vi "Test Switch Tables 2.vi"() -> ()   [LabVIEW 2019]
uses:
  src/LV-Data.PG/LV-Data.PGSQL.lvclass
  <vilib>/addons/_JKI Toolkits/Caraya/classes/Test/Test.lvclass
  <vilib>/addons/_JKI Toolkits/Caraya/classes/Assert/Assert.lvclass
  <vilib>/addons/_JKI Toolkits/Caraya/classes/Assert/Assert Not Error.vi
panel:
  out "error out":errorcluster
  in  "error in (no error)":errorcluster
  out "Data.PG out":refnum<class "LV-Data.PGSQL.lvclass">
  in  "Data.PG":refnum<class "LV-Data.PGSQL.lvclass">
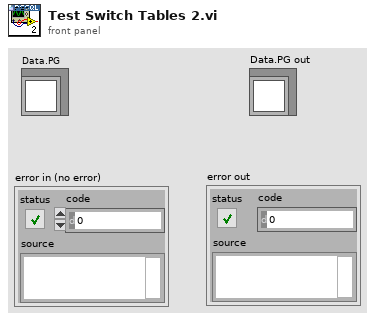
[diagram p1: front panel]
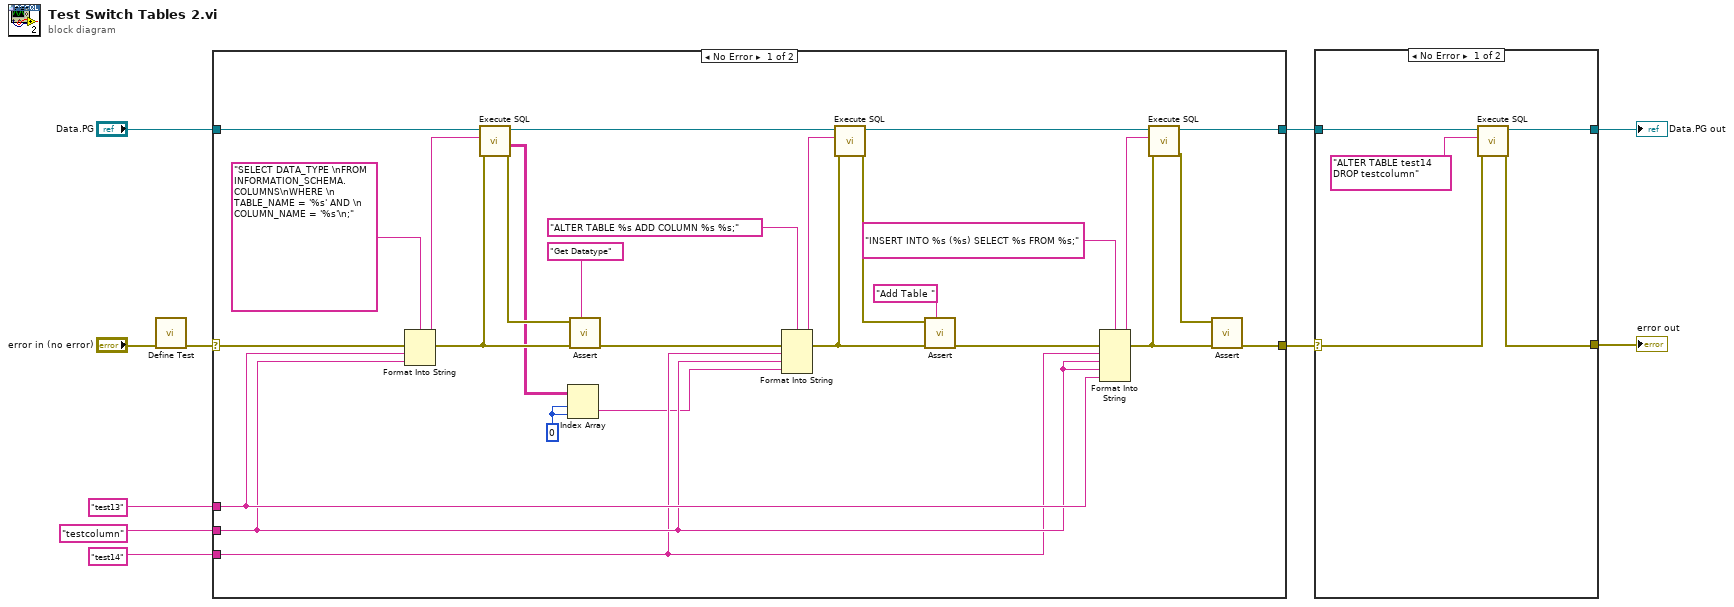
[diagram p0: block diagram]
diagram:
  n1 = call <vilib>:"Define Test.vi"("error in (no error)"="error in (no error)") -> ("error out"=w2:errorcluster)  [unwired: 9 in, 1 out]
  n2 = case shown="No Error" w2 {
    selector: w2 -> [w24 w39]
    tunnel: "test14" ("Old Column") -> [w26 _]
    tunnel: "testcolumn" ("Old Column") -> [w27 _]
    tunnel: "Data.PG" -> [w25 w40]
    tunnel: [w38 w40] -> w4
    tunnel: "test13" ("Old Table") -> [w28 _]
    tunnel: [w17 w39] -> w3
    frame No Error {
      w32 = 0 ("index (row)")
      n3 = Format Into String(format string="SELECT DATA_TYPE \nFROM INFORMATION_SCHEMA.COLUMNS\nWHERE \n     TABLE_NAME = '%s' AND \n     COLUMN_NAME = '%s'\n;", error in=w24, w28, w27) -> (resulting string=w29:string, error out=w14:errorcluster)  [unwired: 1 in]
      n4 = call "Execute SQL.vi"("error in"=w14, "SQL"=w29, "LV-Data.PGSQL"=w25) -> ("error out"=w13:errorcluster, "Result"=w11:string[][], "LV-Data.PGSQL out"=w34:refnum<class "LV-Data.PGSQL.lvclass">)  [unwired: 5 in, 1 out]
      n5 = Index Array(array=w11, index (row)=w32, index (col)=w32) -> (element=w12:string)
      n6 = call-poly <vilib>:"Assert.vi"("Label"="Get Datatype", "error in (no error)"=w14, "Not Error?"=w13) -> ("error out"=w23:errorcluster)  [unwired: 7 in, 1 out]
      n7 = Format Into String(format string="ALTER TABLE %s ADD COLUMN %s %s;", error in=w23, w26, w27, w12) -> (resulting string=w35:string, error out=w15:errorcluster)  [unwired: 1 in]
      n8 = call "Execute SQL.vi"("error in"=w15, "SQL"=w35, "LV-Data.PGSQL"=w34) -> ("error out"=w20:errorcluster, "LV-Data.PGSQL out"=w33:refnum<class "LV-Data.PGSQL.lvclass">)  [unwired: 5 in, 2 out]
      n9 = call-poly <vilib>:"Assert.vi"("Label"="Add Table ", "error in (no error)"=w15, "Not Error?"=w20) -> ("error out"=w21:errorcluster)  [unwired: 7 in, 1 out]
      n10 = Format Into String(format string="INSERT INTO %s (%s) SELECT %s FROM %s;", error in=w21, w26, w27, w27, w28) -> (resulting string=w30:string, error out=w16:errorcluster)  [unwired: 1 in]
      n11 = call "Execute SQL.vi"("error in"=w16, "SQL"=w30, "LV-Data.PGSQL"=w33) -> ("error out"=w18:errorcluster, "LV-Data.PGSQL out"=w38:refnum<class "LV-Data.PGSQL.lvclass">)  [unwired: 5 in, 2 out]
      n12 = call-poly <vilib>:"Assert.vi"("error in (no error)"=w16, "Not Error?"=w18) -> ("error out"=w17:errorcluster)  [unwired: 8 in, 1 out]
    }
    frame Error {
    }
  }
  n13 = case shown="No Error" w3 {
    selector: w3 -> [w41 w47]
    tunnel: [w44 w47] -> w6
    tunnel: [w45 w46] -> w5
    tunnel: w4 -> [w42 w46]
    frame No Error {
      n14 = call "Execute SQL.vi"("error in"=w41, "SQL"="ALTER TABLE test14 DROP testcolumn", "LV-Data.PGSQL"=w42) -> ("error out"=w44:errorcluster, "LV-Data.PGSQL out"=w45:refnum<class "LV-Data.PGSQL.lvclass">)  [unwired: 5 in, 2 out]
    }
    frame Error {
    }
  }
  "Data.PG out" <- w5
  "error out" <- w6
